vi "List-Item Name From ID and Name .vi"(7 "Separate Sign":string="-", 9 "Name":string, 10 "ID":i64=123456789, 11 "List":refnum<vi>) -> (3 "List Out":refnum<vi>)   [LabVIEW 2024]
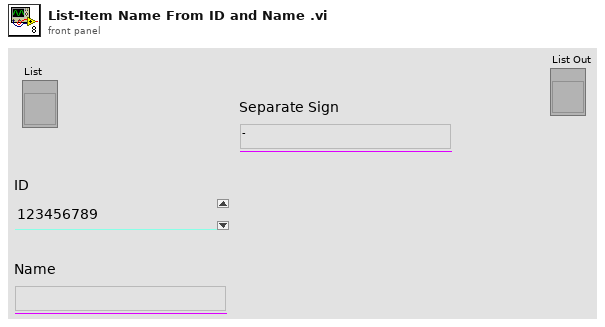
[diagram p1: front panel]
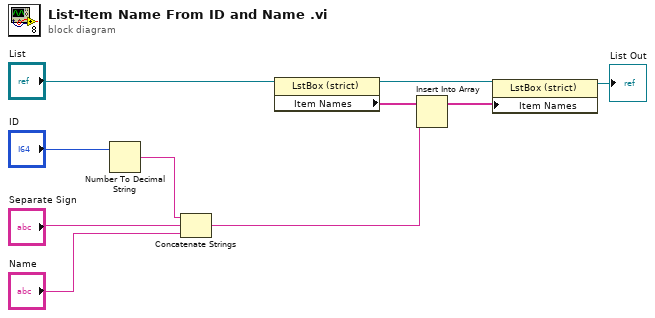
[diagram p0: block diagram]
diagram:
  n1 = Number To Decimal String(number="ID") -> (decimal integer string=w9:string)  [unwired: 1 in]
  n2 = Concatenate Strings(w9, "Separate Sign", "Name") -> (w2:string)
  n3 = property class="LstBox (strict)"(reference="List") -> (reference out=w4:refnum<vi>, "Item Names"=w5:string[])  [unwired: 1 in, 1 out]
  n4 = Insert Into Array(array=w5, new element=w2) -> (w3:string[])  [unwired: 1 in]
  n5 = property class="LstBox (strict)"(reference=w4, "Item Names"=w3) -> (reference out=→"List Out":refnum<vi>)  [unwired: 1 in, 1 out]
